vi "ExSubCreateFileDisplayMultImage.vi"(0 "Camera Handle":u32, 1 "Pulser Handle":u32, 2 "File and Display Name":string, 3 "error in (no error)":errorcluster, 4 "Number of Images":u32=1 min=1 step=1) -> (5 "Handles Out":T1, 6 "Array":u32[](array[numeric]), 7 "error out":errorcluster)   [LabVIEW 2010]
panel:
  # "ExSubCreateFileDisplayMultImage.vi:\nThis is a SubVI that creates a file, display and image objects and returns the handles bundled in a cluster that includes a pulser and camera handle"
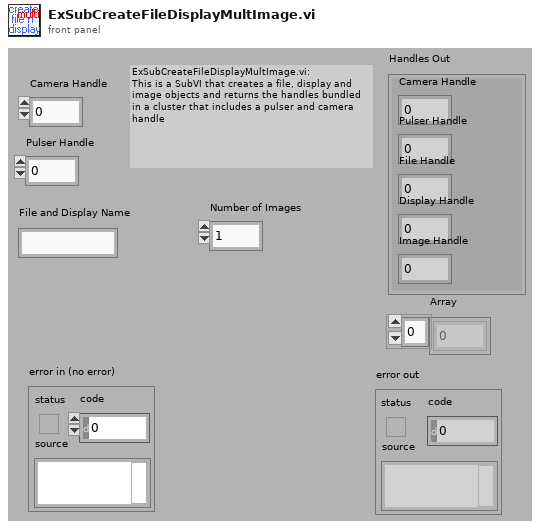
[diagram p1: front panel]
types:
  T1 = cluster{"Camera Handle":u32, "Pulser Handle":u32, "File Handle":u32, "Display Handle":u32, "Image Handle":u32}
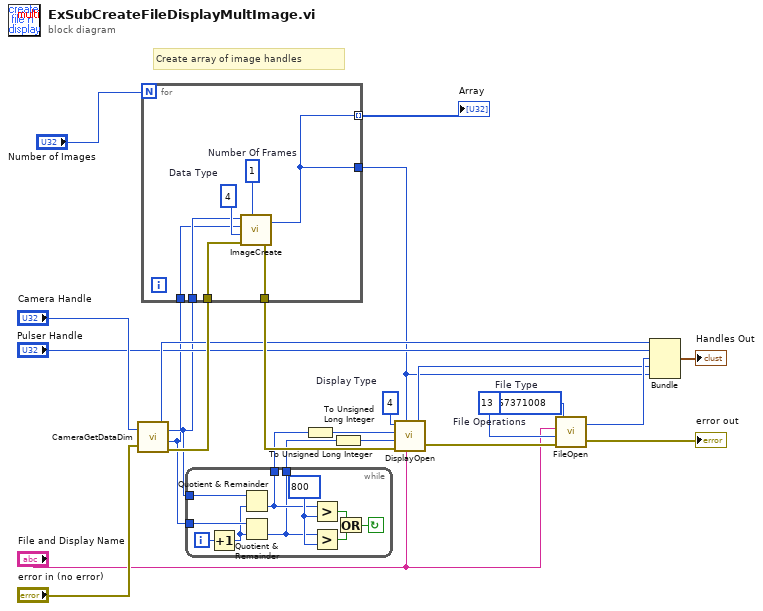
[diagram p0: block diagram]
diagram:
  w9 = u32 4  # Display Type
  w11 = 13  # File Operations
  w12 = 67371008  # File Type
  # "Create array of image handles"
  n1 = call <userlib>:"CameraGetDataDim.vi"("Camera Handle"="Camera Handle", "error in"="error in (no error)") -> ("Camera Handle"=w18:u32, "Xdim"=w8:u32, "Ydim"=w7:u32, "error out"=w24:errorcluster)
  n2 = for {
    N: "Number of Images" -> [_]
    tunnel: w24 -> [w31]
    tunnel: [w30] -> w23
    tunnel: [w29] -> w14
    tunnel: w8 -> [w26]
    tunnel: w7 -> [w25]
    tunnel: [w29] -> w1 mode=indexing
    w27 = u32 1  # Number Of Frames
    w28 = u32 4  # Data Type
    n3 = call <userlib>:"ImageCreate.vi"("X dimension"=w26, "Y dimension"=w25, "Data Type"=w28, "error in"=w31, "Number Of Frames"=w27) -> ("Image Handle"=w29:u32, "error out"=w30:errorcluster)
  }
  "Array" <- w1
  n4 = while {
    tunnel: w8 -> [w40]
    tunnel: w7 -> [w39]
    tunnel: [w34] -> w6
    tunnel: [w33] -> w5
    i -> [w38]
    stop <- w35 continue-if-true
    w41 = 800
    n5 = Increment(x=w38) -> (x+1=w32:i32)
    n6 = Quotient & Remainder(x=w40, y=w32) -> (floor(x/y)=w34:u32)  [unwired: 1 out]
    n7 = Quotient & Remainder(x=w39, y=w32) -> (floor(x/y)=w33:u32)  [unwired: 1 out]
    n8 = Greater?(x=w34, y=w41) -> (0:w37:bool)
    n9 = Greater?(x=w33, y=w41) -> (0:w36:bool)
    n10 = Or(x=w37, y=w36) -> (x .or. y?=w35:bool)
  }
  n11 = To Unsigned Long Integer(number=w6) -> (unsigned 32bit integer=w4:u32)
  n12 = To Unsigned Long Integer(number=w5) -> (unsigned 32bit integer=w3:u32)
  n13 = call <userlib>:"DisplayOpen.vi"("Display Title"="File and Display Name", "Image Handle"=w14, "error in"=w23, "Display Height"=w3, "Display Width"=w4, "Display Type"=w9) -> ("error out"=w22:errorcluster, "Display Handle"=w15:u32)
  n14 = call <userlib>:"FileOpen.vi"("error in"=w22, "File Operations"=w11, "FileName"="File and Display Name", "File Type"=w12) -> ("error out"=→"error out":errorcluster, "File Handle"=w16:u32)
  n15 = Bundle("Camera Handle"=w18, "Pulser Handle"="Pulser Handle", "File Handle"=w16, "Display Handle"=w15, "Image Handle"=w14) -> (→"Handles Out":T1)  [unwired: 1 in]
